vi "Read Config File.vi"(8 "error in (no error)":errorcluster, 11 "Config_Read in":refnum<class "Config_Read_BML.lvclass">) -> (0 "error out":errorcluster, 3 "Config_Read out":refnum<class "Config_Read_BML.lvclass">)   [LabVIEW 2018, in "Config_Read_BML.lvclass"]
uses:
  Config_Read_BML.lvclass
  <vilib>/Utility/file.llb/Read Delimited Spreadsheet (string).vi
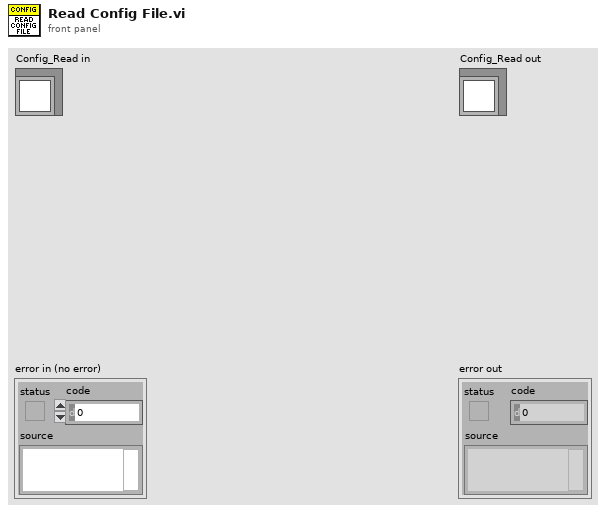
[diagram p1: front panel]
types:
  T1 = typedef "Config_Read_BML.lvclass/Frame_Data.ctl" = cluster{"Pattern_Name":string, "Operation Mode":T2, "BurstLength":T3, "FSN":u8, "Start_Addr":u16, "Data":u8[], "R/W?":T4, "Opcode":string[], "ChipID":u8, "num of wait cycle of read":i8}
  T2 = typedef "Config_Read_BML.lvclass/OperationMode.ctl" = enum8{"Normal", "ImmeEffect", "InitSlaveID", "LoadData"}
  T3 = typedef "Config_Read_BML.lvclass/BurstLength.ctl" = enum8{"0", "2", "3", "4", "5", "8", "16", "32"}
  T4 = typedef "Config_Read_BML.lvclass/RW_Option.ctl" = enum16{"Read", "Write", "R/W"}
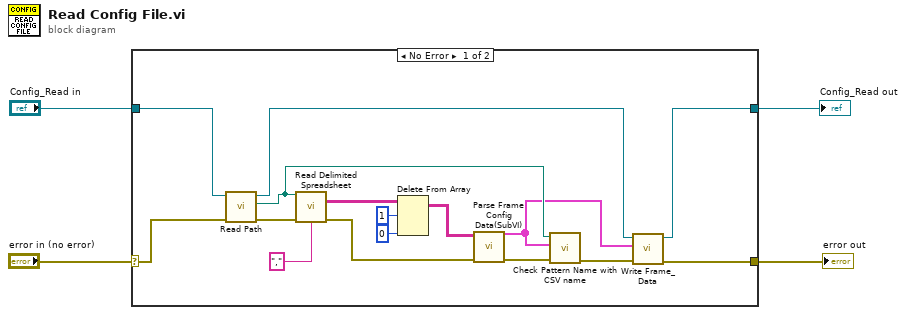
[diagram p0: block diagram]
diagram:
  n1 = case shown="No Error" "error in (no error)" {
    selector: "error in (no error)" -> [w19 w22]
    tunnel: [w9 w22] -> w3
    tunnel: [w10 w21] -> w1
    tunnel: "Config_Read in" -> [w20 w21]
    frame No Error {
      n2 = call-dynamic "Read Path.vi"("error in (no error)"=w19, "Config_Read in"=w20) -> ("error out"=w18:errorcluster, "Path"=w6:path, "Config_Read out"=w11:refnum<class "Config_Read_BML.lvclass">)  [unwired: 7 in]
      n3 = call-poly <vilib>:"Read Delimited Spreadsheet.vi"("file path (dialog if empty)"=w6, "error in (no error)"=w18, "delimiter (\\t)"="," ("delimiter (\\t)")) -> ("all rows"=w16:string[][], "error out"=w12:errorcluster)  [unwired: 7 in, 4 out]
      n4 = Delete From Array(array=w16, length=1, index (row)=0) -> (array with subset deleted=w13:string[][])  [unwired: 1 in, 1 out]
      n5 = call "Parse Frame Config Data(SubVI).vi"("error in (no error)"=w12, "all rows"=w13) -> ("error out"=w8:errorcluster, "Data Array out"=w5:T1[])  [unwired: 8 in]
      n6 = call "Check Pattern Name with CSV name.vi"("error in (no error)"=w8, "Data Array out"=w5, "Path"=w6) -> ("error out"=w7:errorcluster)  [unwired: 8 in]
      n7 = call-dynamic "Write Frame_Data.vi"("error in (no error)"=w7, "FRM_Data_Array"=w5, "Config_Read in"=w11) -> ("error out"=w9:errorcluster, "Config_Read out"=w10:refnum<class "Config_Read_BML.lvclass">)  [unwired: 7 in]
    }
    frame Error {
    }
  }
  "error out" <- w3
  "Config_Read out" <- w1
